vi "Set Duty Cycle.vi"(8 "Error In":errorcluster, 10 "Duty Cycles":T1[](array[typedef]), 11 "LINX Device Config":T2) -> (0 "Error Out":errorcluster, 3 "LINX Device Config":T2)   [LabVIEW 2011, in "LVH-LINX.lvlib" / "Device.lvlib"]
doc: "Set the duty cycle of the specified PWM channels. A duty cylce of 0 is fully off while a duty cylce of 255 is fully on. A duty cycle of 127 is 50% on."
uses:
  Device.lvlib
  Type Defs/LINX Device Config.ctl
  Type Defs/Interface.ctl
  Type Defs/TCP Config.ctl
  Type Defs/Device Family.ctl
  Type Defs/Peripherals/PWM/PWM Duty Cycle Control.ctl
  Type Defs/Error Type.ctl
  LVH-LINX.lvlib
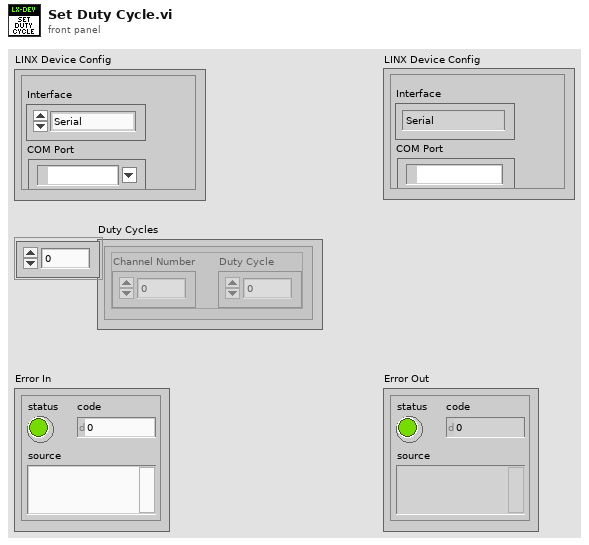
[diagram p1: front panel]
types:
  T1 = typedef "LVH-LINX.lvlib/PWM Duty Cycle Control.ctl" = cluster{"Channel Number":u8, "Duty Cycle":u8}
  T2 = typedef "LVH-LINX.lvlib/Device.lvlib/LINX Device Config.ctl" = cluster{"Interface":T3, "COM Port":refnum<visa-resource-name>, "TCP Configuration":T4, "Device Family":T5, "Device ID":u8, "Device Name":string, "TCP Ref":refnum<k5>}
  T3 = typedef "LVH-LINX.lvlib/Interface.ctl" = enum16{"Serial", "TCP"}
  T4 = typedef "LVH-LINX.lvlib/Device.lvlib/TCP Config.ctl" = cluster{"IP Address":string, "Port":u16}
  T5 = typedef "LVH-LINX.lvlib/Device Family.ctl" = enum8{"National Instruments", "Digilent", "Arduino"}
  T6 = typedef "LVH-LINX.lvlib/Error Type.ctl" = enum16{"Unknown", "Timeout", "Corrupt Return Packet", "Unable To Connect", "Command Not Supported", "Channel DNE"}
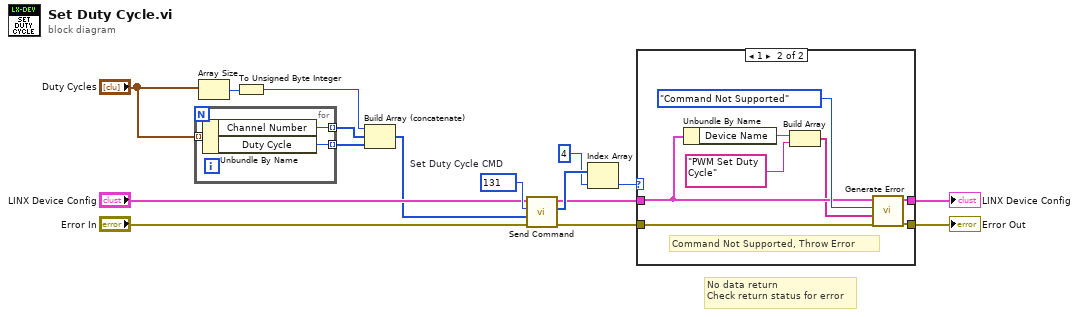
[diagram p0: block diagram]
diagram:
  w15 = u16 131  # Set Duty Cycle CMD
  # "No data return\nCheck return status for error"
  n1 = for {
    tunnel: "Duty Cycles" -> [w19] mode=indexing
    tunnel: [w18] -> w13 mode=indexing
    tunnel: [w17] -> w1 mode=indexing
    n2 = Unbundle By Name(w19) -> ("Channel Number"=w18:u8, "Duty Cycle"=w17:u8)
  }
  n3 = Array Size(array="Duty Cycles") -> (size(s)=w12:i32)
  n4 = To Unsigned Byte Integer(number=w12) -> (unsigned 8bit integer=w11:u8)
  n5 = Build Array (concatenate)(w11, w13, w1) -> (w10:u8[])
  n6 = call "Send Command.vi"("Error In"="Error In", "ARGS"=w10, "CMD"=w15, "LINX Device Config"="LINX Device Config") -> ("Error Out"=w3:errorcluster, "Response"=w9:u8[], "LINX Device Config"=w5:T2)  [unwired: 5 in]
  n7 = Index Array(array=w9, index=4) -> (element=w7:u8)
  n8 = case shown="1" w7 {
    tunnel: [w21 w27] -> w6
    tunnel: w5 -> [w21 w23]
    tunnel: [w20 w28] -> w4
    tunnel: w3 -> [w20 w29]
    frame 0, Default {
      # "Status OK"
    }
    frame 1 {
      # "Command Not Supported, Throw Error"
      n9 = Unbundle By Name(w23) -> ("Device Name"=w25:string)
      n10 = Build Array(w25, "PWM Set Duty Cycle") -> (w22:string[])
      n11 = call "Generate Error.vi"("Error In"=w29, "Arguments"=w22, "Error Type"=Error_Type."Command Not Supported", "LINX Device Config"=w23) -> ("Error Out"=w28:errorcluster, "LINX Device Config"=w27:T2)  [unwired: 6 in]
    }
  }
  "Error Out" <- w4
  "LINX Device Config" <- w6
